vi "Register Front Panel.vi"(8 "error in (no error)":errorcluster, 9 "menu ref":refnum<k9>, 10 "This VI":refnum<vi>, 11 "DAQMan in":refnum<class "Cfg Grandmaster.lvclass">) -> (0 "error out":errorcluster, 2 "Event Registration Refnum":refnum<event-registration>, 3 "DAQMan out":refnum<class "Cfg Grandmaster.lvclass">)   [LabVIEW 2012, in "Configuration Grandmaster.lvlib" / "Cfg Grandmaster.lvclass"]
uses:
  Cfg Grandmaster.lvclass
  Common/Controls/Group Timing Info.ctl
  Common/Controls/LS Lock Sizes.ctl
  Actor Nest/Class Actor Nest/Actor Nest.lvclass/Actor Nest.ctl
  Class FP Ctrls/FP Controls.lvclass/FP Controls.ctl
  Cfg Grandmaster.lvclass/Cfg Grandmaster.ctl
  Class FP Ctrls/Read Init UI.vi
  Class FP Ctrls/Read HS Timing.vi
  Class FP Ctrls/Read LS Timing.vi
  Class FP Ctrls/Read Active Chassis.vi
  Class FP Ctrls/Read Update HS Bcklg.vi
  Class FP Ctrls/Read Update LS Bcklg.vi
  Class FP Ctrls/Read Error Count.vi
  Class FP Ctrls/Read Lock to LS.vi
  Actor Nest/Class Actor Nest/Read Shutdown.vi
  Class FP Ctrls/FP Controls.lvclass
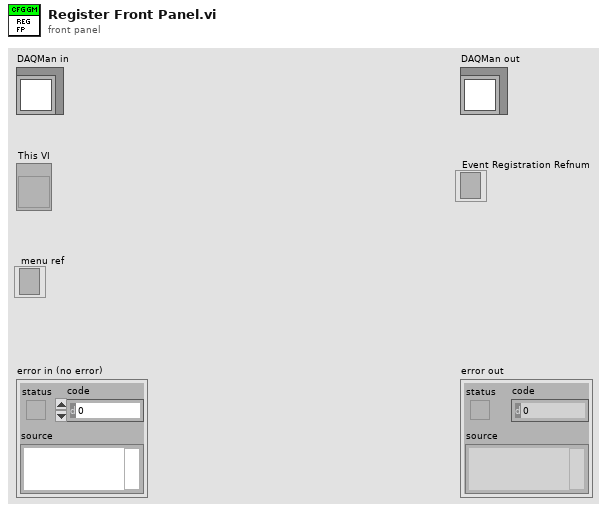
[diagram p1: front panel]
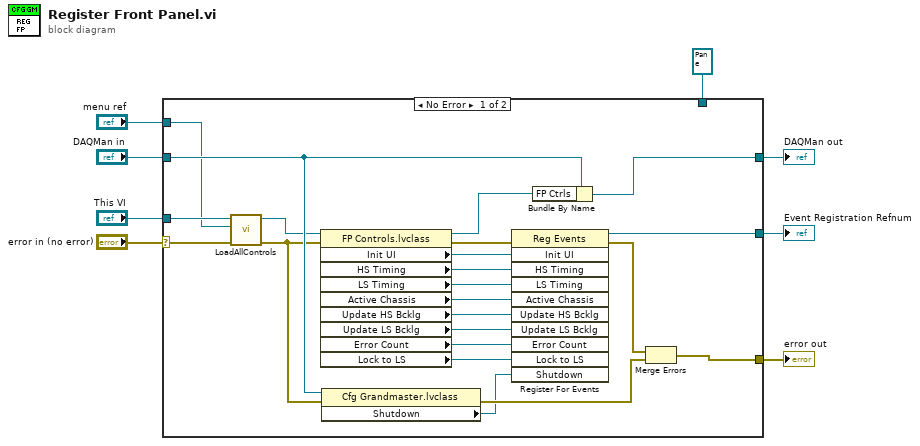
[diagram p0: block diagram]
diagram:
  n1 = case shown="No Error" "error in (no error)" {
    selector: "error in (no error)" -> [w19 w33]
    tunnel: [w22 w33] -> w7
    tunnel: [w20 w32] -> w5
    tunnel: "DAQMan in" -> [w21 w32]
    tunnel: [w25 w31] -> w2
    tunnel: "This VI" -> [w16 _]
    tunnel: "menu ref" -> [w15 _]
    tunnel: refnum<event-registration> refnum ("Event Registration Refnum") -> [_ w31]
    frame No Error {
      n2 = call "LoadAllControls.vi"("error in (no error)"=w19, "menu reference"=w15, "This VI"=w16) -> ("error out"=w18:errorcluster, "FP Controls out"=w14:refnum<class "FP Controls.lvclass">)  [unwired: 7 in]
      n3 = property class="FP Controls.lvclass"(reference=w14, error in=w18) -> (reference out=w17:refnum<class "FP Controls.lvclass">, error out=w26:errorcluster, "Init UI"=w30:refnum<user-event>, "HS Timing"=w29:refnum<user-event>, "LS Timing"=w28:refnum<user-event>, "Active Chassis"=w27:refnum<user-event>, "Update HS Bcklg"=w12:refnum<user-event>, "Update LS Bcklg"=w11:refnum<user-event>, "Error Count"=w13:refnum<user-event>, "Lock to LS"=w9:refnum<user-event>)
      n4 = property class="Cfg Grandmaster.lvclass"(reference=w21, error in=w18) -> (error out=w23:errorcluster, "Shutdown"=w10:refnum<user-event>)  [unwired: 1 out]
      n5 = register-events(error in=w26, w30, w29, w28, w27, w12, w11, w13, w9, w10) -> (reference out=w25:refnum<event-registration>, error out=w24:errorcluster)  [unwired: 1 in]
      n6 = Bundle By Name(cluster=w21, "FP Ctrls"=w17) -> (w20:refnum<class "Cfg Grandmaster.lvclass">)
      n7 = Merge Errors(w24, w23) -> (w22:errorcluster)
    }
    frame Error {
    }
  }
  "error out" <- w7
  "DAQMan out" <- w5
  "Event Registration Refnum" <- w2
